vi "SP SP - click.vi"(8 "error in (no error)":errorcluster, 11 "JSON string":string) -> (0 "error out":errorcluster, 3 "value":string)   [LabVIEW 2020, in "ui-testing.lvlib"]
doc: "copyright: Thomas Zilliox©"
uses:
  ui-testing.lvlib
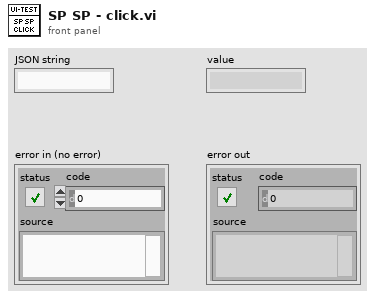
[diagram p1: front panel]
types:
  T1 = cluster{"control":string, "subpanel":string, "subsubpanel":string}
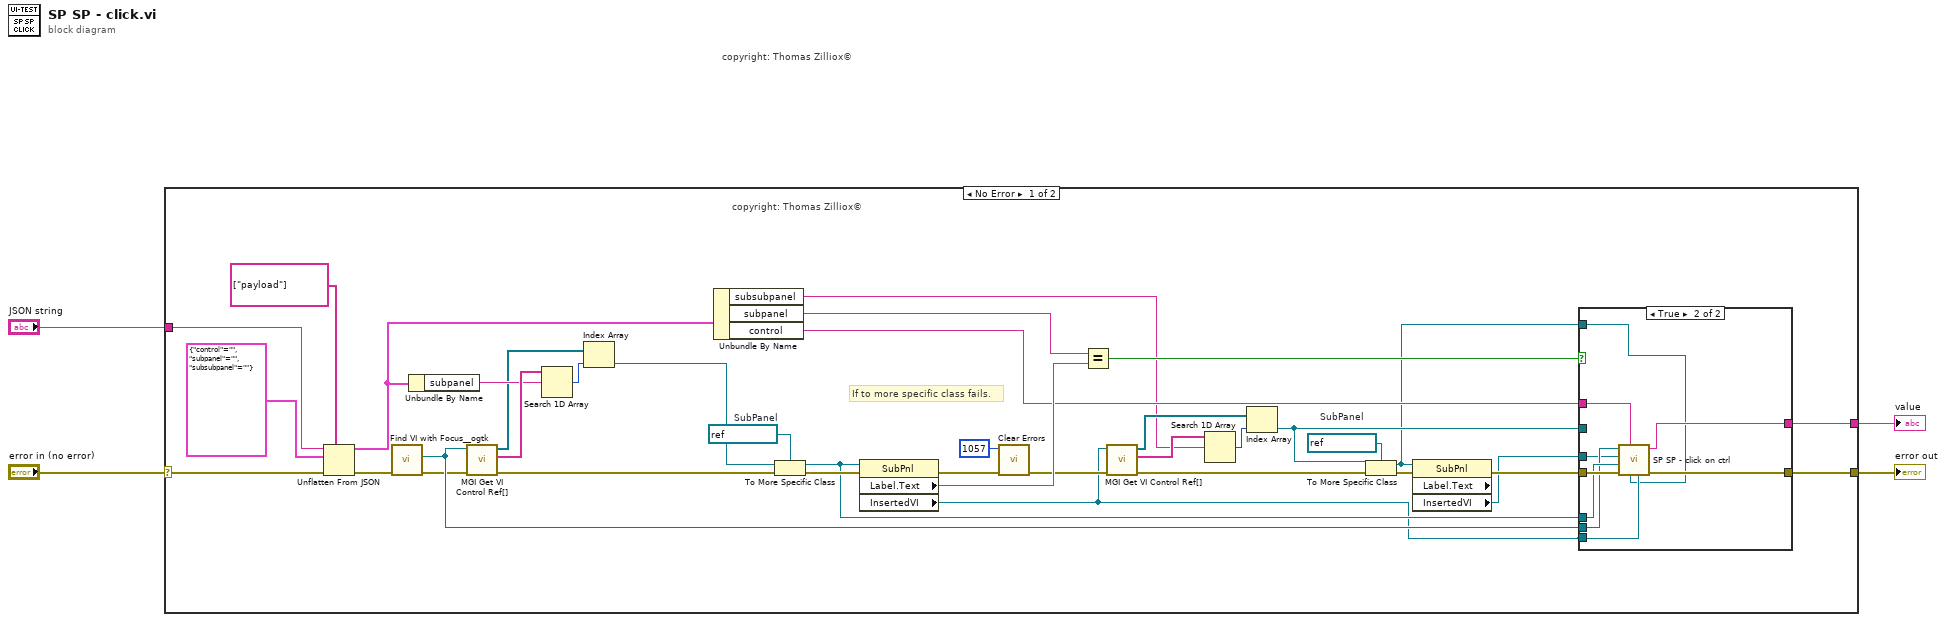
[diagram p0: block diagram]
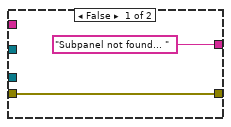
[diagram p2: hidden frame]
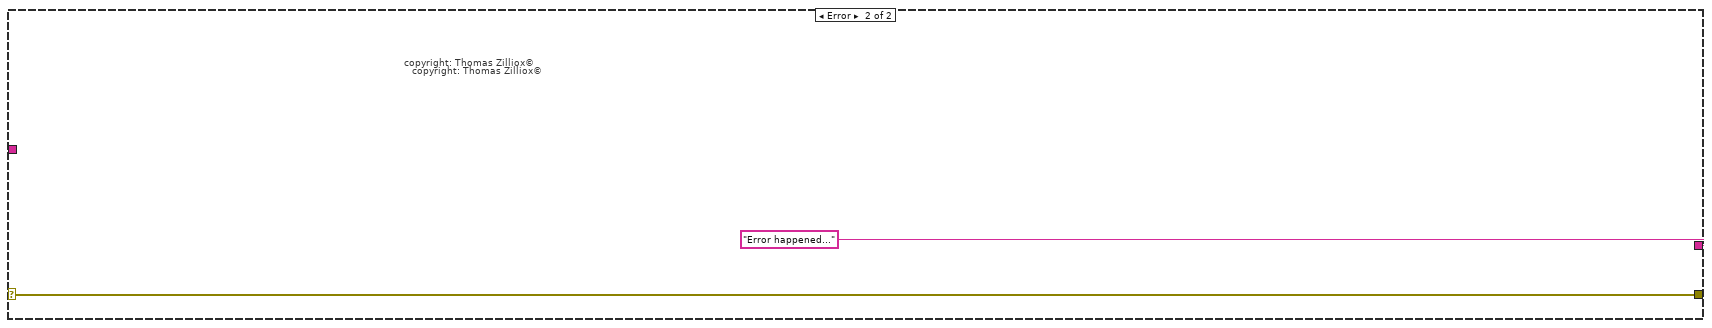
[diagram p3: hidden frame]
diagram:
  # "copyright: Thomas Zilliox©"
  n1 = case shown="No Error" "error in (no error)" {
    selector: "error in (no error)" -> [w38 w55]
    tunnel: "JSON string" -> [w40 _]
    tunnel: [w39 w55] -> w3
    tunnel: [w36 "Error happened..."] -> w1
    frame No Error {
      w11 = refnum<vi> refnum  # SubPanel
      w18 = refnum<vi> refnum  # SubPanel
      # "If to more specific class fails."
      # "copyright: Thomas Zilliox©"
      n2 = Unflatten From JSON(path=string[] ["payload"], JSON string=w40, type and defaults=T1 {"control"="", "subpanel"="", "subsubpanel"=""}, error in (no error)=w38) -> (value=w32:T1, error out=w41:errorcluster)  [unwired: 3 in]
      n3 = call <userlib>:"Find VI with Focus__ogtk.vi"("error in"=w41) -> ("error out"=w34:errorcluster, "VI with Focus"=w35:refnum<vi>)  [unwired: 6 in, 3 out]
      n4 = Unbundle By Name(w32) -> ("subpanel"=w31:string)
      n5 = call <userlib>:"MGI Get VI Control Ref[].vi"("error in"=w34, "VI (Caller)"=w35) -> ("error out"=w28:errorcluster, "Control Label Chain[i]"=w33:string[], "Control[i]"=w30:refnum<vi>[])  [unwired: 6 in, 1 out]
      n6 = Search 1D Array(1D array=w33, element=w31) -> (index of element=w29:i32)  [unwired: 1 in]
      n7 = Index Array(array=w30, index=w29) -> (element=w27:refnum<vi>)
      n8 = Unbundle By Name(w32) -> ("subsubpanel"=w13:string, "subpanel"=w26:string, "control"=w24:string)
      n9 = To More Specific Class(target class=w18, reference=w27, error in=w28) -> (specific class reference=w17:refnum<vi>, error out=w19:errorcluster)
      n10 = property class="SubPnl"(reference=w17, error in=w19) -> (error out=w22:errorcluster, "Label.Text"=w25:string, "InsertedVI"=w6:refnum<vi>)  [unwired: 1 out]
      n11 = call <vilib>:"Clear Errors.vi"("error in (no error)"=w22, "specific error code to clear (0: all)"=1057) -> ("error out"=w20:errorcluster)  [unwired: 4 in, 1 out]
      n12 = Equal?(x=w26, y=w25) -> (x = y?=w23:bool)
      n13 = call <userlib>:"MGI Get VI Control Ref[].vi"("error in"=w20, "VI (Caller)"=w6) -> ("error out"=w9:errorcluster, "Control Label Chain[i]"=w14:string[], "Control[i]"=w15:refnum<vi>[])  [unwired: 6 in, 1 out]
      n14 = Search 1D Array(1D array=w14, element=w13) -> (index of element=w16:i32)  [unwired: 1 in]
      n15 = Index Array(array=w15, index=w16) -> (element=w10:refnum<vi>)
      n16 = To More Specific Class(target class=w11, reference=w10, error in=w9) -> (specific class reference=w5:refnum<vi>, error out=w8:errorcluster)
      n17 = property class="SubPnl" props=["Label", "Text", "InsertedVI"](reference=w5, error in=w8) -> (error out=w12:errorcluster, "InsertedVI"=w7:refnum<vi>)  [unwired: 2 out]
      n18 = case shown="True" w23 {
        tunnel: [w44 w51] -> w39
        tunnel: w12 -> [w44 w53]
        tunnel: w24 -> [_ w50]
        tunnel: ["Subpanel not found... " ("result string") w52] -> w36
        tunnel: w35 -> [_ w48]
        tunnel: w17 -> [_ w49]
        tunnel: w10 -> [_ _]
        tunnel: w7 -> [_ w47]
        tunnel: w6 -> [_ w46]
        tunnel: w5 -> [_ w45]
        frame False {
        }
        frame True {
          n19 = call "SP SP - click on ctrl.vi"("subVI caller"=w46, "subsubpanel"=w45, "Control Label"=w50, "error in (no error)"=w53, "subpanel"=w49, "subVI"=w47, "VI with Focus"=w48) -> ("error out"=w51:errorcluster, "return value"=w52:string)  [unwired: 3 in]
        }
      }
    }
    frame Error {
      # "copyright: Thomas Zilliox©"
      # "copyright: Thomas Zilliox©"
    }
  }
  "error out" <- w3
  "value" <- w1
